vi "UIM Executable Build Localization.vi"() -> ()   [LabVIEW 2020]
doc: "This example visualizes a way to specify plugins in code. This makes it easier to build executables that use the UIM API."
uses:
  Plugin UIPs/CaptionUIP/CaptionUIP.lvclass
  C:/GitHub/LabVIEW-User-Interface-Manager/UIP Interface/UIP Interface.lvclass
  Plugin UIPs/DisabledUIP/DisabledUIP.lvclass
  Plugin UIPs/DescriptionUIP/DescriptionUIP.lvclass
  Plugin UIPs/PositionUIP/PositionUIP.lvclass
  Plugin UIPs/SizeUIP/SizeUIP.lvclass
  Plugin UIPs/TipStripUIP/TipStripUIP.lvclass
  Plugin UIPs/VisibleUIP/VisibleUIP.lvclass
  UIM Class/UIM.lvclass
panel:
  in  "Boolean":bool
  out "Waveform Chart":dbl(graph)
  in  "File Path Control":path
  in  "Numeric Control":dbl
  in  "String":string
  in  "Stop Button":bool
  in  "UI State":u16(ring) items=["English", "Polski"]
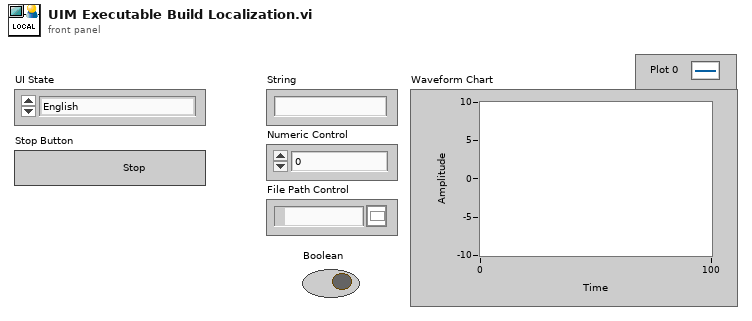
[diagram p1: front panel]
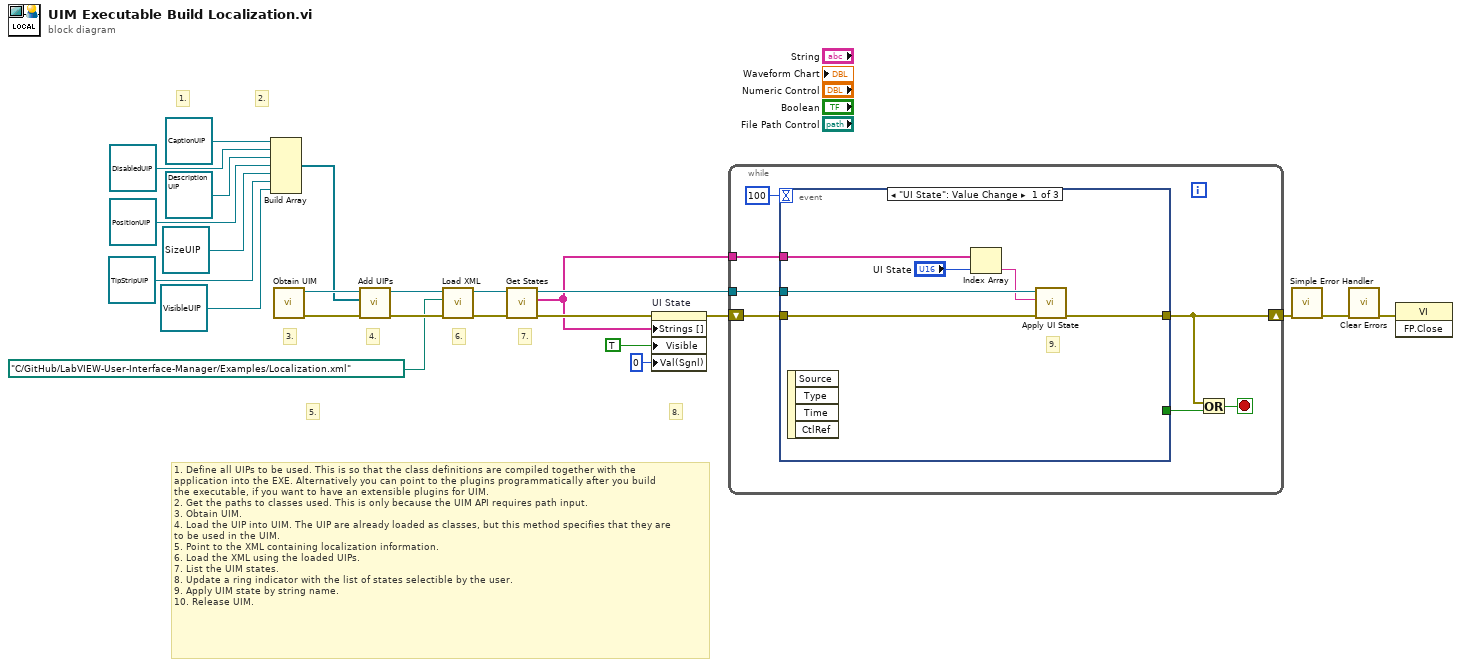
[diagram p0: block diagram]
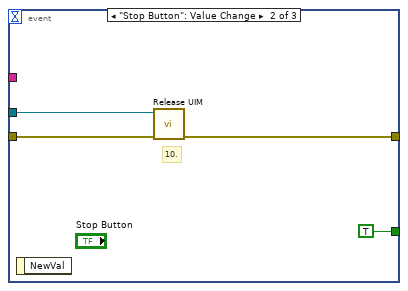
[diagram p2: hidden frame]
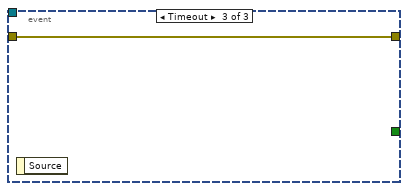
[diagram p3: hidden frame]
diagram:
  # "1. Define all UIPs to be used. This is so that the class definitions are compiled together with the\napplication into the EXE. Alternatively you can point to the plugins programmatically after you build\nthe executable, if you want to have an extensible plugins for UIM.\n2. Get the paths to classes used. This is only because the UIM API requires path input.\n3. Obtain UIM.\n4. Load the UIP into UIM. The UIP are already loaded as classes, but this method specifies that they are\nto be used in the UIM.\n5. Point to the XML containing localization information.\n6. Load the XML using the loaded UIPs.\n7. List the UIM states.\n8. Update a ring indicator with the list of states selectible by the user.\n9. Apply UIM state by string name.\n10. Release UIM."
  # "8."
  # "7."
  # "6."
  # "5."
  # "4."
  # "3."
  # "2."
  # "1."
  n1 = Build Array(refnum<class "CaptionUIP.lvclass"> refnum ("CaptionUIP.lvclass"), refnum<class "DisabledUIP.lvclass"> refnum ("DisabledUIP.lvclass"), refnum<class "DescriptionUIP.lvclass"> refnum ("DescriptionUIP.lvclass"), refnum<class "PositionUIP.lvclass"> refnum ("PositionUIP.lvclass"), refnum<class "SizeUIP.lvclass"> refnum ("SizeUIP.lvclass"), refnum<class "TipStripUIP.lvclass"> refnum ("TipStripUIP.lvclass"), refnum<class "VisibleUIP.lvclass"> refnum ("VisibleUIP.lvclass")) -> (w2:refnum<class "UIP Interface.lvclass">[])
  n2 = call "Obtain UIM.vi"() -> ("Error Out"=w13:errorcluster, "UIM Handle"=w15:refnum<data-value>)  [unwired: 10 in]
  n3 = call "Add UIPs.vi"("Error In"=w13, "UIPs"=w2, "UIM In"=w15) -> ("Error Out"=w14:errorcluster, "UIM Out"=w12:refnum<data-value>)  [unwired: 7 in]
  n4 = call "Load XML.vi"("Error In"=w14, "XML File"=path "C:/GitHub/LabVIEW-User-Interface-Manager/Examples/Localization.xml", "UIM In"=w12) -> ("Error Out"=w18:errorcluster, "UIM Out"=w21:refnum<data-value>)  [unwired: 7 in]
  n5 = call "Get States.vi"("Error In"=w18, "UIM In"=w21) -> ("Error Out"=w19:errorcluster, "States"=w17:string[], "UIM Out"=w20:refnum<data-value>)  [unwired: 7 in]
  n6 = property on="UI State" class="Ring (strict)"(error in=w19, "Strings []"=w17, "Visible"=TRUE, "Val(Sgnl)"=u16 0 ("Value (Signaling)")) -> (error out=w24:errorcluster)  [unwired: 1 in, 1 out]
  n7 = while {
    tunnel: w20 -> [w31]
    tunnel: w17 -> [w29]
    shift-right: [w26] -> w16
    shift-left: w24 -> [w30]
    stop <- w27 stop-if-true
    n8 = event shown="[0] \"UI State\": Value Change" {
      selector: _ -> [_ _ _]
      dyn-events: _ -> [_ _ _]
      timeout: 100 -> [_ _ _]
      tunnel: w31 -> [w37 w40 _]
      tunnel: [_ TRUE _] -> w28
      tunnel: w30 -> [w36 w39 w42]
      tunnel: [w35 w38 w42] -> w26
      tunnel: w29 -> [w32 _ _]
      event "UI State": Value Change {
        # "9."
        n9 = event-data() -> ()  [unwired: 1 in, 4 out]
        n10 = Index Array(array=w32, index="UI State") -> (element=w33:string)
        n11 = call "Apply UI State.vi"("Error In"=w36, "State Name"=w33, "UIM In"=w37) -> ("Error Out"=w35:errorcluster)  [unwired: 7 in, 1 out]
      }
      event "Stop Button": Value Change {
        # "10."
        n12 = event-data() -> ()  [unwired: 1 in, 1 out]
        n13 = call "Release UIM.vi"("Error In"=w39, "UIM Handle"=w40) -> ("Error Out"=w38:errorcluster)  [unwired: 9 in]
      }
      event Timeout {
        n14 = event-data() -> ()  [unwired: 1 in, 1 out]
      }
    }
    n15 = Or(x=w26, y=w28) -> (x .or. y?=w27:bool)
  }
  n16 = call <vilib>:"Simple Error Handler.vi"("error in (no error)"=w16) -> ("error out"=w4:errorcluster)  [unwired: 4 in, 4 out]
  n17 = call <vilib>:"Clear Errors.vi"("error in (no error)"=w4) -> ("error out"=w3:errorcluster)  [unwired: 5 in, 1 out]
  n18 = invoke class="VI" method="FP.Close"(error in=w3) -> ()  [unwired: 2 in, 3 out]
